vi "i2c_write.vi"(4 "Num read":u8, 6 "Bus":u8, 8 "error in":errorcluster, 9 "Data":u8[](array[numeric]) format="%x", 10 "Address":u8, 11 "I2C interface":T1) -> (0 "error out":errorcluster, 1 "Empty Elements Remaining":u32)   [LabVIEW 2014]
uses:
  i2c_interface.ctl
  fpga_reference.ctl
  Common/i2c_command.ctl
  <vilib>/Utility/error.llb/Error Cluster From Error Code.vi
  <vilib>/rvi/errors/niLvFpgaAdjustHostInterfaceError.vi
  <vilib>/rvi/interface/nirviMethod/nirviMethod.xnode
  FPGA Bitfiles/i2cmuxdemux.lvbitx
  <vilib>/FPGAPlugInAG/PCIe-7842R/niLvFpga_WriteFifo_PCIe-7842R.vi
  <vilib>/rvi/errors/niLvFpgaMergeErrorWithErrorCode.vi
panel:
  # "Send a write command to the specified I2C bus and address.  Data is the data to write.  If the FIFO is full then this VI will block until the data can be accepted.\n\nIf \"Num read\" is greater than 0, then send a read command to read the specified number of bytes right after the write command. \n\nFinally, we send send an I2C stop command to release the bus afterwards."
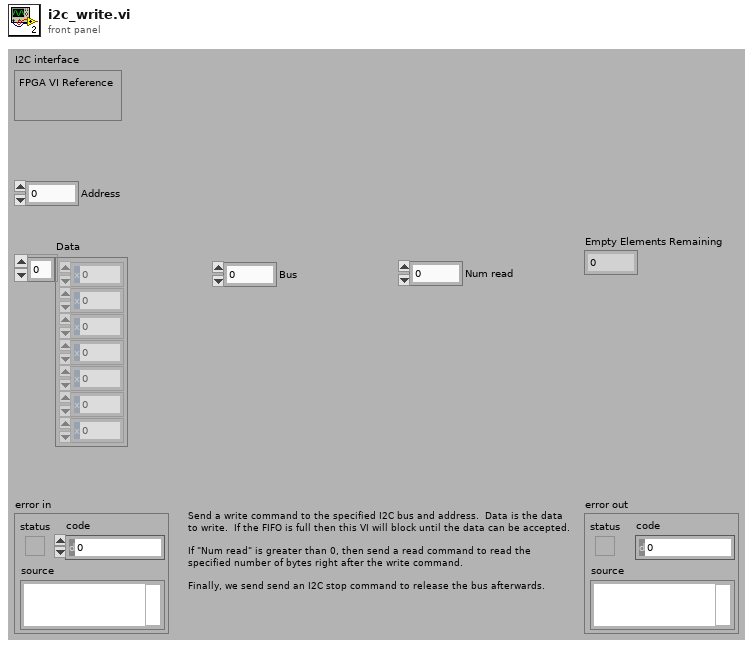
[diagram p1: front panel]
types:
  T1 = typedef "i2c_interface.ctl" = cluster{"FPGA VI Reference":T2}
  T2 = typedef "fpga_reference.ctl" = refnum<k20>
  T3 = typedef "i2c_command.ctl" = enum8{"invalid", "start_write", "start_read", "stop", "sequence"}
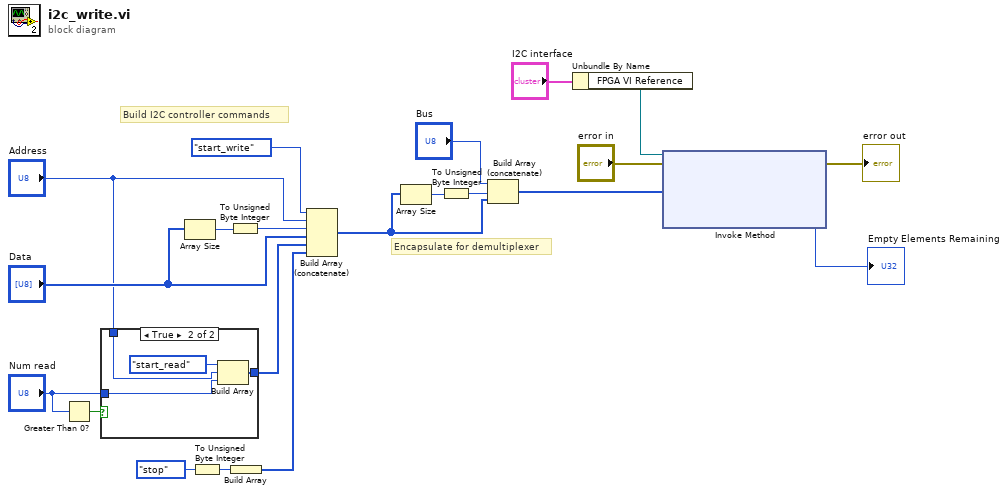
[diagram p0: block diagram]
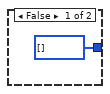
[diagram p2: hidden frame]
diagram:
  # "Build I2C controller commands"
  # "Encapsulate for demultiplexer"
  n1 = Greater Than 0?(x="Num read") -> (x > 0?=w4:bool)
  n2 = case shown="True" w4 {
    tunnel: "Num read" -> [_ w24]
    tunnel: "Address" -> [_ w25]
    tunnel: [u8[] [] w23] -> w1
    frame False {
    }
    frame True {
      n3 = Build Array(i2c_command."start_read" ("Command"), w25, w24) -> (w23:u8[])
    }
  }
  n4 = Array Size(array="Data") -> (size(s)=w20:i32)
  n5 = To Unsigned Byte Integer(number=i2c_command."stop" ("Command")) -> (unsigned 8bit integer=w5:u8)
  n6 = To Unsigned Byte Integer(number=w20) -> (unsigned 8bit integer=w19:u8)
  n7 = Build Array(w5) -> (w13:u8[])
  n8 = Build Array (concatenate)(i2c_command."start_write" ("Command"), "Address", w19, "Data", w1, w13) -> (w10:u8[])
  n9 = Array Size(array=w10) -> (size(s)=w11:i32)
  n10 = To Unsigned Byte Integer(number=w11) -> (unsigned 8bit integer=w9:u8)
  n11 = Build Array (concatenate)("Bus", w9, w10) -> (w7:u8[])
  n12 = Unbundle By Name("I2C interface") -> ("FPGA VI Reference"=w17:T2)
  n13 = xnode "Invoke Method"("FPGA VI Reference In"=w17, "error in"="error in", "Data"=w7) -> ("error out"=→"error out":errorcluster, "Empty Elements Remaining"=→"Empty Elements Remaining":u32)  [unwired: 1 in, 1 out]
